vi "ep_Filter Parameter Calculation.vi"(6 "fs after decimation [Hz]":dbl, 8 "error in (no error)":errorcluster, 9 "fs [Hz]":dbl, 10 "maximum frequency [Hz]":dbl, 11 "filter for frequency measurement":T2={"enable filter? (T)"=TRUE, "passband edge frequency [Hz]"=0.0, "passband ripple [dB]"=0.1, "stopband edge frequency [Hz]"=0.0, "stopband attenuation [dB]"=60.0}) -> (0 "error out":errorcluster, 3 "filter parameters":T1, 5 "total group delay [s]":dbl)   [LabVIEW 2013, in "NI_EP_Power Measurement.lvlib"]
uses:
  <vilib>/addons/Electrical Power/Power Measurement/NI_EP_Power Measurement.lvlib
  <vilib>/addons/Electrical Power/Power Measurement/subVIs/ep_Filter Design.ctl
  <vilib>/Analysis/3filter.llb/Filter Passband Type.ctl
  <vilib>/Analysis/NI_AALBase.lvlib
  <vilib>/addons/Electrical Power/PQ/Resampling/NI_EP_Resample_Host.lvlib
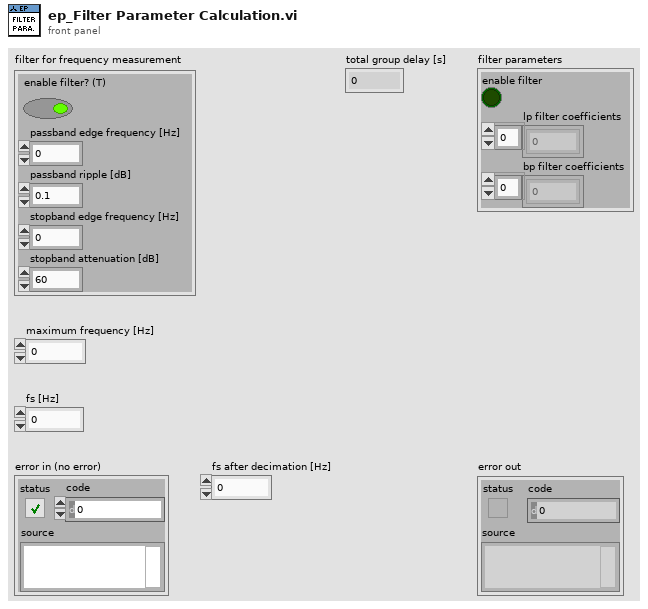
[diagram p1: front panel]
types:
  T1 = cluster{"enable filter":bool, "lp filter coefficients":dbl[], "bp filter coefficients":dbl[]}
  T2 = typedef "NI_EP_Power Measurement.lvlib/ep_Filter Design.ctl" = cluster{"enable filter? (T)":bool, "passband edge frequency [Hz]":dbl, "passband ripple [dB]":dbl, "stopband edge frequency [Hz]":dbl, "stopband attenuation [dB]":dbl}
  T3 = cluster{"fpass 1":dbl, "fstop 1":dbl, "fpass 2 ":dbl, "fstop 2":dbl}
  T4 = cluster{"passband":dbl, "stopband":dbl, "dB/linear? (T: dB)":bool}
  T5 = typedef "NI_AALBase.lvlib/Filter Passband Type.ctl" = enum32{"Lowpass", "Highpass", "Bandpass", "Bandstop"}
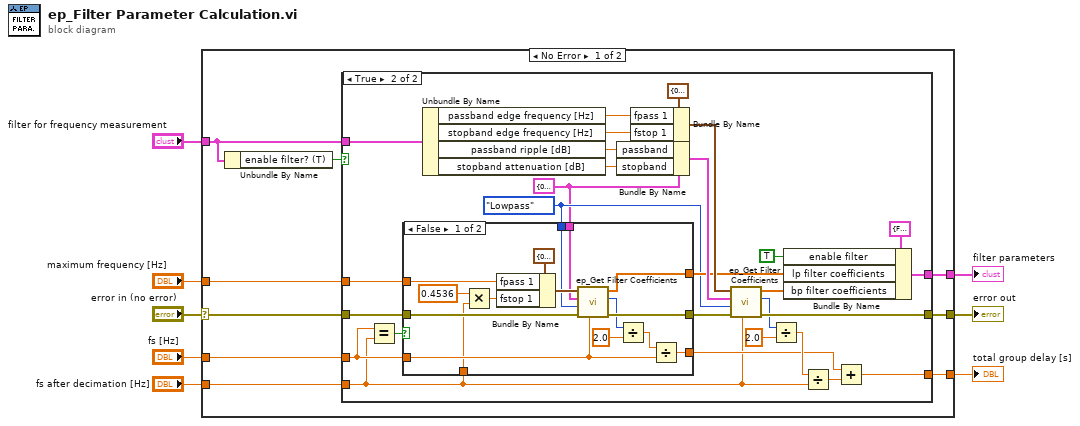
[diagram p0: block diagram]
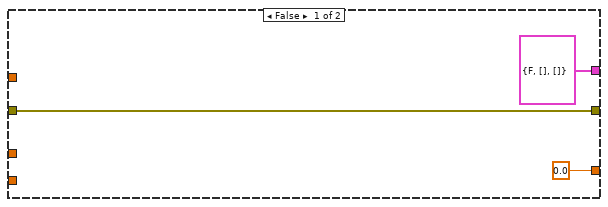
[diagram p2: hidden frame]
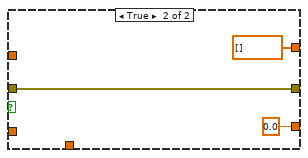
[diagram p3: hidden frame]
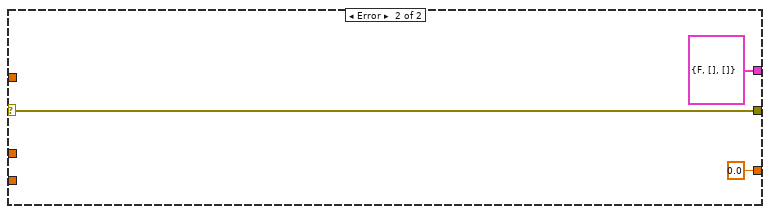
[diagram p4: hidden frame]
diagram:
  n1 = case shown="No Error" "error in (no error)" {
    selector: "error in (no error)" -> [w15 w70]
    tunnel: "filter for frequency measurement" -> [w17 _]
    tunnel: "fs [Hz]" -> [w14 _]
    tunnel: "maximum frequency [Hz]" -> [w13 _]
    tunnel: "fs after decimation [Hz]" -> [w12 _]
    tunnel: [w11 0.0] -> w3
    tunnel: [w10 T1 {"enable filter"=FALSE, "lp filter coefficients"=[], "bp filter coefficients"=[]} ("filter parameters")] -> w2
    tunnel: [w9 w70] -> w1
    frame No Error {
      n2 = Unbundle By Name(w17) -> ("enable filter? (T)"=w16:bool)
      n3 = case shown="True" w16 {
        tunnel: w17 -> [_ w48]
        tunnel: w15 -> [w20 w40]
        tunnel: [w20 w39] -> w9
        tunnel: w13 -> [_ w38]
        tunnel: w14 -> [_ w22]
        tunnel: w12 -> [_ w21]
        tunnel: [0.0 w31] -> w11
        tunnel: [T1 {"enable filter"=FALSE, "lp filter coefficients"=[], "bp filter coefficients"=[]} ("filter parameters") w27] -> w10
        frame False {
        }
        frame True {
          w23 = T4 {"passband"=0.1, "stopband"=60.0, "dB/linear? (T: dB)"=TRUE} ("ripple specs")
          w24 = Filter_Passband_Type."Lowpass" ("filter type")
          n4 = Equal?(x=w22, y=w21) -> (x = y?=w25:bool)
          n5 = case shown="False" w25 {
            tunnel: [w64 w66] -> w47
            tunnel: w40 -> [w63 w66]
            tunnel: w38 -> [w62 _]
            tunnel: w22 -> [w54 _]
            tunnel: w21 -> [w53 _]
            tunnel: [w52 0.0] -> w32
            tunnel: [w51 dbl[] [] ("filter coefficients")] -> w28
            tunnel: w24 -> [w50 _]
            tunnel: w23 -> [w49 _]
            frame False {
              n6 = Multiply(x=0.4536, y=w53) -> (x*y=w61:dbl)
              n7 = Bundle By Name(cluster=T3 {"fpass 1"=0.2, "fstop 1"=0.3, "fpass 2 "=0.0, "fstop 2"=0.0} ("freq specs [Hz]"), "fpass 1"=w62, "fstop 1"=w61) -> (w59:T3)
              n8 = call <vilib>:"ep_Get Filter Coefficients.vi"("fs [Hz]"=w54, "error in (no error)"=w63, "filter type"=w50, "ripple specs"=w49, "freq specs [Hz]"=w59) -> ("error out"=w64:errorcluster, "estimated order"=w57:i32, "filter coefficients"=w51:dbl[])  [unwired: 4 in]
              n9 = Divide(x=w57, y=2.0) -> (x/y=w55:dbl)
              n10 = Divide(x=w55, y=w54) -> (x/y=w52:dbl)
            }
            frame True {
            }
          }
          n11 = Unbundle By Name(w48) -> ("passband edge frequency [Hz]"=w43:dbl, "stopband edge frequency [Hz]"=w42:dbl, "passband ripple [dB]"=w44:dbl, "stopband attenuation [dB]"=w45:dbl)
          n12 = Bundle By Name(cluster=w23, "passband"=w44, "stopband"=w45) -> (w46:T4)
          n13 = Bundle By Name(cluster=T3 {"fpass 1"=0.2, "fstop 1"=0.3, "fpass 2 "=0.0, "fstop 2"=0.0} ("freq specs [Hz]"), "fpass 1"=w43, "fstop 1"=w42) -> (w41:T3)
          n14 = call <vilib>:"ep_Get Filter Coefficients.vi"("fs [Hz]"=w21, "error in (no error)"=w47, "filter type"=w24, "ripple specs"=w46, "freq specs [Hz]"=w41) -> ("error out"=w39:errorcluster, "estimated order"=w34:i32, "filter coefficients"=w29:dbl[])  [unwired: 4 in]
          n15 = Divide(x=w34, y=2.0) -> (x/y=w36:dbl)
          n16 = Bundle By Name(cluster=T1 {"enable filter"=FALSE, "lp filter coefficients"=[], "bp filter coefficients"=[]} ("filter parameters"), "enable filter"=TRUE, "lp filter coefficients"=w28, "bp filter coefficients"=w29) -> (w27:T1)
          n17 = Divide(x=w36, y=w21) -> (x/y=w33:dbl)
          n18 = Add(x=w32, y=w33) -> (x+y=w31:dbl)
        }
      }
    }
    frame Error {
    }
  }
  "filter parameters" <- w2
  "total group delay [s]" <- w3
  "error out" <- w1
